vi "String suchen.vi"(9 "Gasname":string="NO2 High 191C (2of2)", 11 "Such-Namen":string[](array[string])=["CO ", "CO%", "CO2 ", "CO2%", "O2 ", "NO ", "NOx", "NO2 191", "NO2 L", "NO2 H", "N2O", "NH3", "HNCO", "H2O%", "Formaldehyde", "Urea", "Propylen", "Diesel", "Ethylen", "CH4", "Ethan", "Acetylen", "Propane", "Butadien", "Acetaldehyd", "Formic", "MeOH", "SO2", "Toluene", "MethylPentan", "Ammonia", "Ethanol", "Toluene", "Acetic", "Acrolein", "MeOH", "Dodecane", "SO3", "H2S", "H2SO4", "m-Xylene", "o-Xylene", "P-XYLENE", "Benzene", "Ethyl Benzene", "HCN", "Propanal", "Temp. Messzelle", "Druck Messzelle", "sBeam@2500", "Konstant 0", "Konstant 50", "Konstant 100", "Schaltschrank", "Filter", "Pumpe", "HL "]) -> (1 "Index":i32, 3 "Gefunden?":bool)   [LabVIEW 2020, in "Gaszuordnung AO.lvlib"]
uses:
  Gaszuordnung AO.lvlib
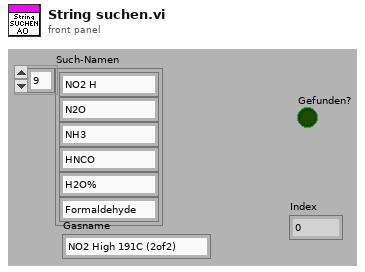
[diagram p1: front panel]
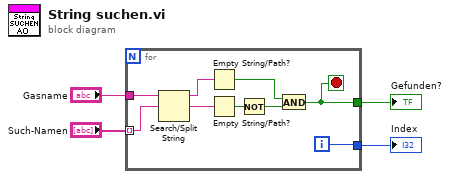
[diagram p0: block diagram]
diagram:
  n1 = for {
    tunnel: "Gasname" -> [w9]
    tunnel: "Such-Namen" -> [w10] mode=indexing
    tunnel: [w5] -> w3
    tunnel: [w11] -> w4
    i -> [w11]
    stop <- w5 stop-if-true
    n2 = Search/Split String(string=w9, search string/char (-)=w10) -> (substring before match=w8:string, match + rest of string=w13:string)  [unwired: 1 in, 1 out]
    n3 = Empty String/Path?(string/path=w8) -> (empty?=w6:bool)
    n4 = Empty String/Path?(string/path=w13) -> (empty?=w12:bool)
    n5 = Not(x=w12) -> (.not. x?=w7:bool)
    n6 = And(x=w6, y=w7) -> (x .and. y?=w5:bool)
  }
  "Index" <- w4
  "Gefunden?" <- w3
